vi "Get_Acceleration.vi"(7 "I2C Channel":u8, 8 "error in (no error)":errorcluster, 11 "LINX Resource In":T2) -> (0 "error out":errorcluster, 2 "XYZ Acceleration(g)":T1, 3 "LINX Resource Out":T2)   [LabVIEW 2014, in "LMH-LINX.lvlib" / "LIS331HH.lvlib"]
doc: "This VI returns acceleration values for each of the axis. The output scaled based on Full Scale selection\n(i.e. @+/- 6g LBs sensitivity is ~3milli-g)\nThe acceleration is output in g's"
uses:
  <vilib>/MakerHub/LINX/Public/Sensors/Accelerometer/LIS331HH/LIS331HH.lvlib
  <vilib>/MakerHub/LINX/LMH-LINX.lvlib
  <vilib>/MakerHub/LINX/Public/Sensors/Accelerometer/LIS331HH/_typeDefs/Register_Map.ctl
  <vilib>/MakerHub/LINX/Public/Sensors/Accelerometer/LIS331HH/Controls/Accelerations.ctl
  <vilib>/MakerHub/LINX/Private/Type Defs/Platform.ctl
  <vilib>/MakerHub/LINX/Private/Type Defs/Interface.ctl
  <vilib>/MakerHub/LINX/Private/Device/Type Defs/TCP Config.ctl
  <vilib>/MakerHub/LINX/Private/Device/Device.lvlib
  <vilib>/MakerHub/LINX/Private/Device/Type Defs/Channels.ctl
  <vilib>/MakerHub/LINX/Private/Device/Type Defs/LINX Device Config.ctl
  <vilib>/MakerHub/LINX/Private/Type Defs/LINX Ref.ctl
panel:
  # "INPUTS"
  # "OUTPUTS"
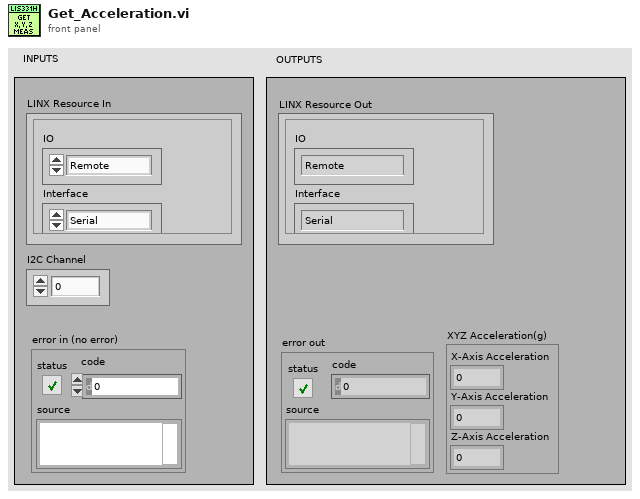
[diagram p1: front panel]
types:
  T1 = cluster{"X-Axis Acceleration":i16, "Y-Axis Acceleration":i16, "Z-Axis Acceleration":i16}
  T2 = typedef "LMH-LINX.lvlib/LINX Ref.ctl" = cluster{"IO":T3, "Interface":T4, "LINX Device Config":T5}
  T3 = typedef "LMH-LINX.lvlib/Platform.ctl" = enum16{"Remote", "Local"}
  T4 = typedef "LMH-LINX.lvlib/Interface.ctl" = enum16{"Serial", "TCP"}
  T5 = typedef "LMH-LINX.lvlib/Device.lvlib/LINX Device Config.ctl" = cluster{"Interface":T4, "COM Port":refnum<visa-resource-name>, "TCP Configuration":T6, "Device Family":u8, "Device ID":u8, "Device Name":string, "TCP Ref":refnum<k5>, "Channels":T7}
  T6 = typedef "LMH-LINX.lvlib/Device.lvlib/TCP Config.ctl" = cluster{"IP Address":string, "Port":u16}
  T7 = typedef "LMH-LINX.lvlib/Channels.ctl" = cluster{"DI":u8[], "DO":u8[], "AI":u8[], "AO":u8[], "PWM":u8[], "QE":u8[], "UART":u8[], "I2C 2":u8[], "SPI":u8[], "CAN":u8[], "Servo":u8[], "AI Ref (V)":dbl, "AI Resolution (Bits)":u8, "AO Ref (V)":dbl, "AO Resolution (Bits)":u8}
  T8 = typedef "Accelerations.ctl" = cluster{"X-Axis Acceleration":sgl, "Y-Axis Acceleration":sgl, "Z-Axis Acceleration":sgl}
  T9 = typedef "LMH-LINX.lvlib/LIS331HH.lvlib/Register_Map.ctl" = u8
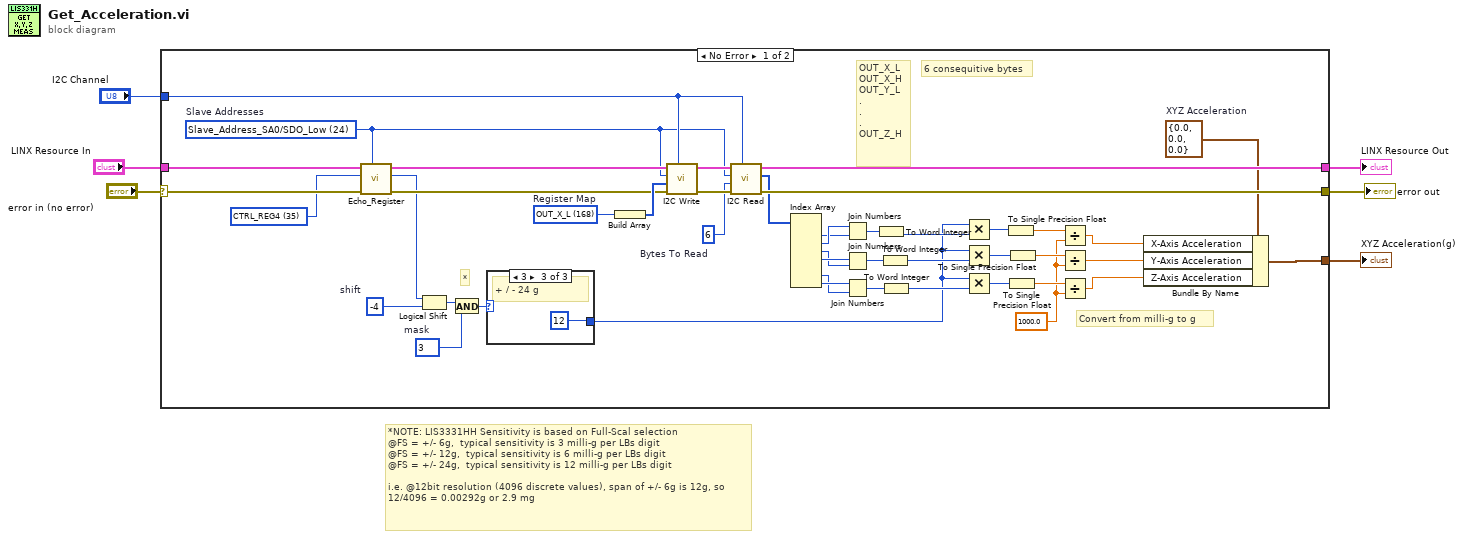
[diagram p0: block diagram]
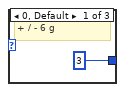
[diagram p2: hidden frame]
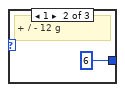
[diagram p3: hidden frame]
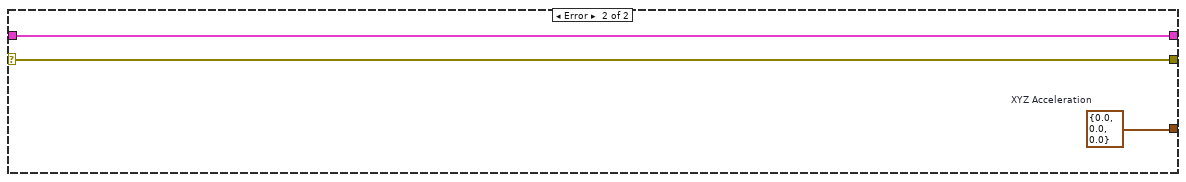
[diagram p4: hidden frame]
diagram:
  # "*NOTE: LIS3331HH Sensitivity is based on Full-Scal selection\n@FS = +/- 6g,  typical sensitivity is 3 milli-g per LBs digit\n@FS = +/- 12g,  typical sensitivity is 6 milli-g per LBs digit\n@FS = +/- 24g,  typical sensitivity is 12 milli-g per LBs digit\n\ni.e. @12bit resolution (4096 discrete values), span of +/- 6g is 12g, so \n12/4096 = 0.00292g or 2.9 mg"
  n1 = case shown="No Error" "error in (no error)" {
    selector: "error in (no error)" -> [w29 w57]
    tunnel: [w46 w57] -> w5
    tunnel: "LINX Resource In" -> [w30 w56]
    tunnel: "I2C Channel" -> [w48 _]
    tunnel: [w35 w56] -> w2
    tunnel: [w39 w55] -> w1
    frame No Error {
      w10 = sgl 1000.0
      w17 = T8 {"X-Axis Acceleration"=0.0, "Y-Axis Acceleration"=0.0, "Z-Axis Acceleration"=0.0}  # XYZ Acceleration
      w23 = i8 3  # mask
      w20 = i8 -4  # shift
      w24 = T9 168 items=["CTRL_REG1"=32, "CTRL_REG2"=33, "CTRL_REG3"=34, "CTRL_REG4"=35, "CTRL_REG5"=36, "HP_FILTER_RESET"=37, "REFERENCE"=38, "STATUS_REG"=39, "OUT_X_L"=168, "OUT_X_H"=41, "OUT_Y_L"=42, "OUT_Y_H"=43, "OUT_Z_L"=44, "OUT_Z_H"=45, "INT1_CFG"=48, "INT1_SOURCE"=49, "INT1_THS"=50, "INT1_DURATION"=51, "INT2_CFG"=52, "INT2_SOURCE"=53, "INT2_THS"=54, "INT2_DURATION"=55]  # Register Map
      w25 = u8 35 items=["CTRL_REG1"=32, "CTRL_REG2"=33, "CTRL_REG3"=34, "CTRL_REG4"=35, "CTRL_REG5"=36, "HP_FILTER_RESET"=37, "REFERENCE"=38, "STATUS_REG"=39, "OUT_X_L"=40, "OUT_X_H"=41, "OUT_Y_L"=42, "OUT_Y_H"=43, "OUT_Z_L"=44, "OUT_Z_H"=45, "INT1_CFG"=48, "INT1_SOURCE"=49, "INT1_THS"=50, "INT1_DURATION"=51, "INT2_CFG"=52, "INT2_SOURCE"=53, "INT2_THS"=54, "INT2_DURATION"=55] ("Register to Echo")
      w47 = u8 6  # Bytes To Read
      w26 = u8 24 items=["Slave_Address_SA0/SDO_Low"=24, "Slave_Address_SA0/SDO_High"=25]  # Slave Addresses
      # "Convert from milli-g to g"
      # "6 consequitive bytes"
      # "*"
      # "OUT_X_L\nOUT_X_H\nOUT_Y_L\n.\n.\n.\nOUT_Z_H"
      n2 = call <vilib>:"Echo_Register.vi"("I2C Channel"=w26, "error in (no error)"=w29, "Register to Echo"=w25, "LINX Resource In"=w30) -> ("error out"=w27:errorcluster, "Register Word"=w19:u8, "LINX Resource Out"=w28:T2)  [unwired: 5 in]
      n3 = Logical Shift(y=w19, x=w20) -> (x << y=w21:i8)
      n4 = And(x=w21, y=w23) -> (x .and. y?=w22:i8)
      n5 = case shown="3" w22 {
        tunnel: [i16 3 ("x") i16 6 ("x") i16 12 ("x")] -> w18
        frame 0, Default {
          # "+ / - 6 g"
        }
        frame 1 {
          # "+ / - 12 g"
        }
        frame 3 {
          # "+ / - 24 g"
        }
      }
      n6 = Build Array(w24) -> (w51:T9[])
      n7 = call <vilib>:"I2C Write.vi"("I2C Channel"=w48, "Error In"=w27, "Data"=w51, "I2C Slave Address (0)"=w26, "LINX Resource"=w28) -> ("Error Out"=w49:errorcluster, "LINX Resource"=w50:T2)  [unwired: 5 in]
      n8 = call <vilib>:"I2C Read.vi"("I2C Channel"=w48, "Error In"=w49, "Bytes To Read"=w47, "I2C Slave Address (0)"=w26, "LINX Resource"=w50) -> ("Error Out"=w46:errorcluster, "Data"=w34:u8[], "LINX Resource"=w35:T2)  [unwired: 4 in]
      n9 = Index Array(array=w34) -> (element #1=w44:u8, element #2=w45:u8, element #3=w42:u8, element #4=w43:u8, element #6=w40:u8, element #7=w41:u8)  [unwired: 7 in, 1 out]
      n10 = Join Numbers(hi=w45, lo=w44) -> ((hi.lo)=w36:u16)
      n11 = Join Numbers(hi=w43, lo=w42) -> ((hi.lo)=w37:u16)
      n12 = Join Numbers(hi=w41, lo=w40) -> ((hi.lo)=w38:u16)
      n13 = To Word Integer(number=w36) -> (16bit integer=w33:i16)
      n14 = To Word Integer(number=w37) -> (16bit integer=w32:i16)
      n15 = To Word Integer(number=w38) -> (16bit integer=w31:i16)
      n16 = Multiply(x=w18, y=w33) -> (x*y=w16:i16)
      n17 = Multiply(x=w18, y=w32) -> (x*y=w14:i16)
      n18 = Multiply(x=w18, y=w31) -> (x*y=w15:i16)
      n19 = To Single Precision Float(number=w16) -> (single precision float=w13:sgl)
      n20 = To Single Precision Float(number=w15) -> (single precision float=w11:sgl)
      n21 = To Single Precision Float(number=w14) -> (single precision float=w12:sgl)
      n22 = Divide(x=w13, y=w10) -> (x/y=w9:sgl)
      n23 = Divide(x=w12, y=w10) -> (x/y=w8:sgl)
      n24 = Divide(x=w11, y=w10) -> (x/y=w7:sgl)
      n25 = Bundle By Name(cluster=w17, "X-Axis Acceleration"=w9, "Y-Axis Acceleration"=w8, "Z-Axis Acceleration"=w7) -> (w39:T8)
    }
    frame Error {
      w55 = T8 {"X-Axis Acceleration"=0.0, "Y-Axis Acceleration"=0.0, "Z-Axis Acceleration"=0.0}  # XYZ Acceleration
    }
  }
  "error out" <- w5
  "LINX Resource Out" <- w2
  "XYZ Acceleration(g)" <- w1
